vi "Multiply.vi"(8 "error in (no error)":errorcluster, 11 "UPNCalculatorAdvanced in":refnum<class "UPNCalculatorAdvanced.lvclass">) -> (0 "error out":errorcluster, 3 "UPNCalculatorAdvanced out":refnum<class "UPNCalculatorAdvanced.lvclass">)   [LabVIEW 2012, in "UPNCalculatorAdvanced Actor.lvlib" / "UPNCalculatorAdvanced.lvclass"]
uses:
  UPNCalculatorAdvanced.lvclass
  UPNCalculator Actor/UPNCalculator/UPNCalculator.lvclass
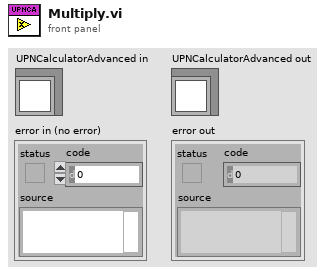
[diagram p1: front panel]
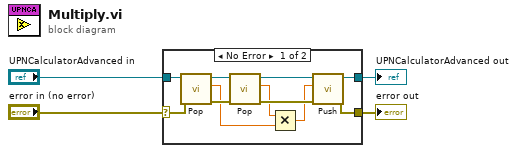
[diagram p0: block diagram]
diagram:
  n1 = case shown="No Error" "error in (no error)" {
    selector: "error in (no error)" -> [w9 w17]
    tunnel: [w8 w17] -> w3
    tunnel: [w10 w16] -> w1
    tunnel: "UPNCalculatorAdvanced in" -> [w15 w16]
    frame No Error {
      n2 = call "Pop.vi"("error in (no error)"=w9, "UPNCalculator in"=w15) -> ("error out"=w14:errorcluster, "Element"=w6:dbl, "UPNCalculator out"=w13:refnum<class "UPNCalculatorAdvanced.lvclass">)  [unwired: 7 in]
      n3 = call "Pop.vi"("error in (no error)"=w14, "UPNCalculator in"=w13) -> ("error out"=w11:errorcluster, "Element"=w7:dbl, "UPNCalculator out"=w12:refnum<class "UPNCalculatorAdvanced.lvclass">)  [unwired: 7 in]
      n4 = Multiply(x=w7, y=w6) -> (x*y=w5:dbl)
      n5 = call "Push.vi"("error in (no error)"=w11, "Element"=w5, "UPNCalculator in"=w12) -> ("error out"=w8:errorcluster, "UPNCalculator out"=w10:refnum<class "UPNCalculatorAdvanced.lvclass">)  [unwired: 7 in]
    }
    frame Error {
    }
  }
  "error out" <- w3
  "UPNCalculatorAdvanced out" <- w1
